vi "V7310.Main-Confirm.vi"(8 "error in":errorcluster) -> (0 "error out":errorcluster)   [LabVIEW 2014]
uses:
  V7310.Action.ctl
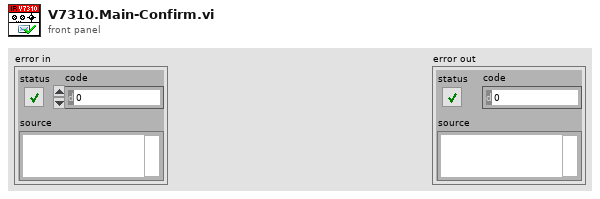
[diagram p1: front panel]
types:
  T1 = typedef "V7310.Action.ctl" = enum32{"idle", "constructor", "destructor", "--- V7310 ---", "Init", "Confirm Msg", "Start", "Stop"}
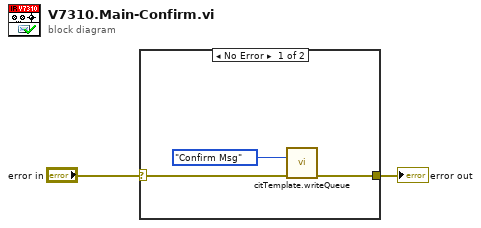
[diagram p0: block diagram]
diagram:
  n1 = case shown="No Error" "error in" {
    selector: "error in" -> [w3 w6]
    tunnel: [w4 w6] -> w1
    frame No Error {
      n2 = call "citTemplate.writeQueue.vi"("event in (if not connected:all statemachine with data event)"=V7310.Action."Confirm Msg" ("Action"), "error in (no error)"=w3) -> ("error out"=w4:errorcluster)  [unwired: 13 in]
    }
    frame Error {
    }
  }
  "error out" <- w1
